vi "byte_stuffing_decod.vi"(3 "String IN":string) -> (0 "bytes DEL":i32, 1 "String OUT":string)   [LabVIEW 2010]
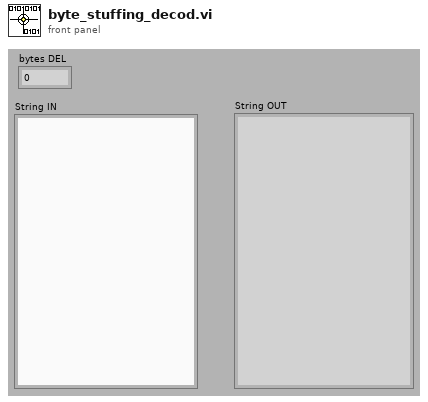
[diagram p1: front panel]
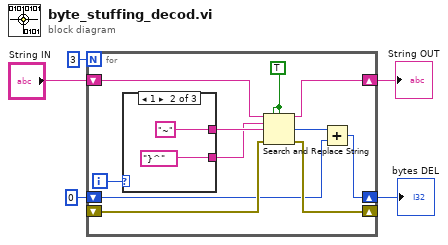
[diagram p0: block diagram]
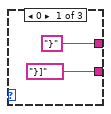
[diagram p2: hidden frame]
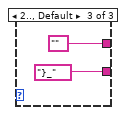
[diagram p3: hidden frame]
diagram:
  n1 = for {
    N: 3 -> [_]
    shift-right: [w16] -> w1
    shift-left: "String IN" -> [w15]
    shift-right: [w13] -> _
    shift-left: _ -> [w12]
    shift-right: [w9] -> w3
    shift-left: 0 -> [w8]
    i -> [w14]
    w10 = TRUE ("ignore case? (F)")
    n2 = case shown="1" w14 {
      tunnel: ["}" "~" ""] -> w7
      tunnel: ["}]" "}^" "}_"] -> w6
      frame 0 {
      }
      frame 1 {
      }
      frame 2.., Default {
      }
    }
    n3 = Search and Replace String(replace all?=w10, case sensitive?=w10, input string=w15, search string=w6, replace string=w7, error in=w12) -> (result string=w16:string, number of replacements=w11:i32, error out=w13:errorcluster)  [unwired: 2 in, 1 out]
    n4 = Add(x=w11, y=w8) -> (x+y=w9:i32)
  }
  "String OUT" <- w1
  "bytes DEL" <- w3
